vi "Pre Launch Init.vi"(11 "WS Test Client in":refnum<class "WS Test Client.lvclass">) -> (0 "error out":errorcluster, 3 "WS Test Client out":refnum<class "WS Test Client.lvclass">)   [LabVIEW 2016, in "WS Full LabVIEW Test.lvlib" / "WS Test Client.lvclass"]
doc: "Sends a high priority message to it's self to notify the monitor that it's spawned. If it's in the runtime environment, this message is never sent, meaning the monitor will never spawn\n\nCopyright: MGI\n\nAuthored by Derek Trepanier\nsupport@mooregoodideas.com\nwww.mooregoodideas.com\n\nCopyright (c) 2014, Moore Good Ideas, Inc.\n\nAll rights reserved.\n\nRedistribution and use in source and binary forms, with or without modification, are permitted provided that the following conditions are met:\n\n * Redistributions of source code must retain the above copyright notice, this list of conditions and the following disclaimer.\n * Redistributions in binary form must reproduce the above copyright notice, this list of conditions and the following disclaimer in the documentation and/or other materials provided with the distribution.\n * Neither the name of Moore Good Ideas, Inc. nor the names of its contributors may be used to endorse or promote products derived from this software without specific prior written permission.\n\nTHIS SOFTWARE IS PROVIDED BY THE COPYRIGHT HOLDERS AND CONTRIBUTORS \"AS IS\" AND ANY EXPRESS OR IMPLIED WARRANTIES, INCLUDING, BUT NOT LIMITED TO, THE IMPLIED WARRANTIES OF MERCHANTABILITY AND FITNESS FOR A PARTICULAR PURPOSE ARE DISCLAIMED. IN NO EVENT SHALL THE COPYRIGHT OWNER OR CONTRIBUTORS BE LIABLE FOR ANY DIRECT, INDIRECT, INCIDENTAL, SPECIAL, EXEMPLARY, OR CONSEQUENTIAL DAMAGES (INCLUDING, BUT NOT LIMITED TO, PROCUREMENT OF SUBSTITUTE GOODS OR SERVICES; LOSS OF USE, DATA, OR PROFITS; OR BUSINESS INTERRUPTION) HOWEVER CAUSED AND ON ANY THEORY OF LIABILITY, WHETHER IN CONTRACT, STRICT LIABILITY, OR TORT (INCLUDING NEGLIGENCE OR OTHERWISE) ARISING IN ANY WAY OUT OF THE USE OF THIS SOFTWARE, EVEN IF ADVISED OF THE POSSIBILITY OF SUCH DAMAGE."
uses:
  WS Test Client.lvclass
  <vilib>/ActorFramework/Message Enqueuer/Message Enqueuer.lvclass
  WS Test Client.lvclass/WS Test Client.ctl
  <vilib>/MGI/Monitored Actor/Monitored Actor/Monitored Actor/Monitored Actor.lvclass
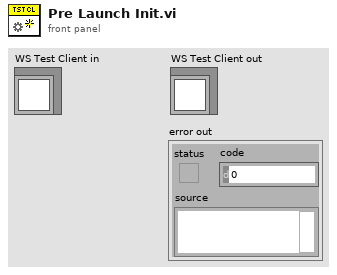
[diagram p1: front panel]
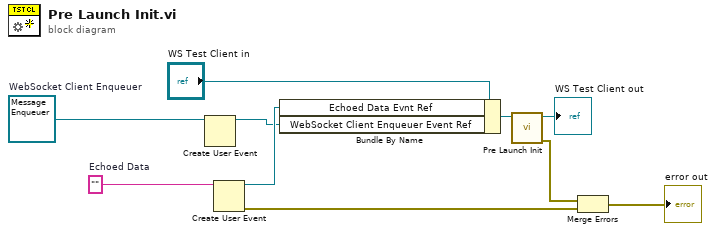
[diagram p0: block diagram]
diagram:
  w2 = refnum<class "Message Enqueuer.lvclass"> refnum  # WebSocket Client Enqueuer
  w7 = ""  # Echoed Data
  n1 = Create User Event(user event datatype=w2) -> (user event=w1:refnum<user-event>)  [unwired: 1 in, 1 out]
  n2 = Create User Event(user event datatype=w7) -> (user event=w5:refnum<user-event>, error out=w3:errorcluster)  [unwired: 1 in]
  n3 = Bundle By Name(cluster="WS Test Client in", "Echoed Data Evnt Ref"=w5, "WebSocket Client Enqueuer Event Ref"=w1) -> (w6:refnum<class "WS Test Client.lvclass">)
  n4 = call-parent "Pre Launch Init.vi"("Monitored Actor in"=w6) -> ("error out"=w10:errorcluster, "Monitored Actor out"=→"WS Test Client out":refnum<class "WS Test Client.lvclass">)  [unwired: 9 in]
  n5 = Merge Errors(w10, w3) -> (→"error out":errorcluster)
